vi "两点的距离.vi"(1 "y2":dbl, 2 "x2":dbl, 3 "y1":dbl, 4 "x1":dbl) -> (0 "de":dbl)   [LabVIEW 2013]
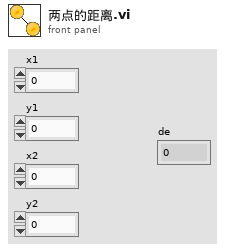
[diagram p1: front panel]
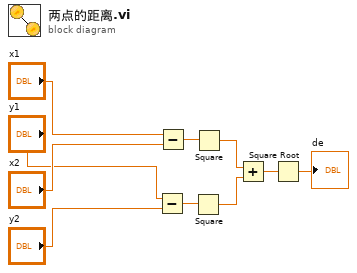
[diagram p0: block diagram]
diagram:
  n1 = Subtract(x="y1", y="y2") -> (x-y=w7:dbl)
  n2 = Subtract(x="x1", y="x2") -> (x-y=w8:dbl)
  n3 = Square(x=w7) -> (x^2=w3:dbl)
  n4 = Square(x=w8) -> (x^2=w4:dbl)
  n5 = Add(x=w4, y=w3) -> (x+y=w2:dbl)
  n6 = Square Root(x=w2) -> (sqrt(x)=→"de":dbl)
